vi "FOCUS_V42.vi"(9 "X-pixels":sgl=256.0, 11 "Run":bool) -> (0 "Retrace pixels":sgl, 10 "Pixel Clock (Hz)":sgl)   [LabVIEW 2010] (continued)
                            n2197 = To Unsigned Byte Integer(number=w3928) -> (unsigned 8bit integer=w3920:u8[])
                            n2198 = Add(x=w3895, y=w3899) -> (x+y=w3904:sgl[])
                            n2199 = To Unsigned Byte Integer(number=w3904) -> (unsigned 8bit integer=w3892:u8[])
                          }
                        }
                      }
                    }
                    n2200 = case shown="True" "Overlay Images" {
                      tunnel: w3665 -> [w4139 w4158]
                      tunnel: [w4139 w4141] -> w3812
                      tunnel: w3664 -> [w4138 w4160]
                      tunnel: [w4138 _] -> w3813
                      frame False {
                      }
                      frame True {
                        n2201 = To Word Integer(number=w4158) -> (16bit integer=w4159:i16[])
                        n2202 = Subtract(x=w4159, y=w4160) -> (x-y=w4140:i16[])
                        n2203 = Add(x=w4159, y=w4160) -> (x+y=w4154:i16[])
                        n2204 = Increment(x=w4154) -> (x+1=w4164:i16[])
                        n2205 = Divide(x=w4140, y=w4164) -> (x/y=w4163:dbl[])
                        n2206 = Absolute Value(x=w4140) -> (abs(x)=w4156:i16[])
                        n2207 = Multiply(x=w4163, y=u8 2) -> (x*y=w4161:dbl[])
                        n2208 = Round To Nearest(number=w4161) -> (nearest integer value=w4147:dbl[])
                        n2209 = Divide(x=w4156, y=2.0) -> (x/y=w4153:dbl[])
                        n2210 = Divide(x=w4154, y=2.0) -> (x/y=w4152:dbl[])
                        n2211 = Add(x=w4153, y=w4152) -> (x+y=w4150:dbl[])
                        n2212 = Divide(x=w4150, y=5.0) -> (x/y=w4149:dbl[])
                        n2213 = Round To Nearest(number=w4149) -> (nearest integer value=w4148:dbl[])
                        n2214 = Multiply(x=5.0 ("y"), y=w4148) -> (x*y=w4146:dbl[])
                        n2215 = Add(x=w4147, y=w4146) -> (x+y=w4145:dbl[])
                        n2216 = Subtract(x=w4145, y=2.0) -> (x-y=w4142:dbl[])
                        n2217 = To Unsigned Byte Integer(number=w4142) -> (unsigned 8bit integer=w4141:u8[])
                      }
                    }
                    n2218 = Greater Or Equal?(x=w3723, y=w3722) -> (x >= y?=w3657:bool)
                    n2219 = Sign(1:w3761) -> (0:w3760:i32)
                    n2220 = local write "Scan Backlock"(w3711) -> ()
                    n2221 = case shown="-1" w3760 {
                      tunnel: "Zoom" -> [_ w3965 w3970]
                      frame 0, Default {
                      }
                      frame 1 {
                        n2222 = Multiply(x=w3965, y=sgl 1.25) -> (x*y=w3963:sgl)
                        n2223 = local write "Zoom"(w3963) -> ()
                      }
                      frame -1 {
                        n2224 = Multiply(x=w3970, y=sgl 0.8) -> (x*y=w3966:sgl)
                        n2225 = Greater Or Equal?(x=w3966, y=sgl 0.28) -> (x >= y?=w3968:bool)
                        n2226 = case shown="True" w3968 {
                          tunnel: w3966 -> [_ w3971]
                          frame False {
                          }
                          frame True {
                            n2227 = local write "Zoom"(w3971) -> ()
                          }
                        }
                      }
                    }
                    n2228 = Not(x=w3680) -> (.not. x?=→"On?":bool)
                    n2229 = case shown="True" w3657 {
                      tunnel: w3769 -> [w3975 w4004]
                      tunnel: [w3975 w4003] -> w3768
                      tunnel: w3767 -> [w3976 w3982]
                      tunnel: [w3976 w3990] -> w3766
                      tunnel: w3718 -> [w3973 w3987]
                      tunnel: w3719 -> [w3974 w3984]
                      tunnel: [w3974 w3985] -> w3721
                      tunnel: [w3973 w3988] -> w3720
                      tunnel: [w3972 w3981] -> w3717
                      tunnel: w3716 -> [w3972 w3980]
                      tunnel: "scattering length [µm]" -> [_ w3977]
                      frame False {
                      }
                      frame True {
                        n2230 = local read "Sutter scale z"() -> (w3978:sgl)
                        n2231 = call "VISA MP-285 Get Z Position.vi"("Input: Duty Cluster"=w4004) -> ("Output: Z axis (microns)"=w4002:sgl, "Output: Duty Cluster"=w4003:T18, "error?"=w3981:bool)
                        n2232 = Multiply(x=w3978, y=w4002) -> (x*y=w3990:sgl)
                        n2233 = Equal?(x=TRUE, y="GetFirst") -> (x = y?=w3994:bool)
                        n2234 = Not Equal?(x="GetFirst", y=w3984) -> (x != y?=w3993:bool)
                        n2235 = Equal?(x=TRUE, y="GetLast") -> (x = y?=w3996:bool)
                        n2236 = Not Equal?(x="GetLast", y=w3987) -> (x != y?=w3998:bool)
                        n2237 = Subtract(x=w3990, y=w3982) -> (x-y=w3999:sgl)
                        n2238 = And(x=w3981, y=w3980) -> (x .and. y?=w3979:bool)
                        n2239 = Not Equal To 0?(x=w3999) -> (x != 0?=w4001:bool)
                        n2240 = Compound Arithmetic op=AND(w3994, w3993, w3979) -> (w3992:bool)
                        n2241 = Compound Arithmetic op=AND(w3979, w3996, w3998) -> (w3991:bool)
                        n2242 = Compound Arithmetic op=AND("IntensityAutomatic", w4001, w3979) -> (w3983:bool)
                        n2243 = case shown="True" w3992 {
                          tunnel: w3990 -> [_ w4007]
                          tunnel: "GetFirst" -> [_ w4006]
                          tunnel: [w4005 w4006] -> w3985
                          tunnel: w3984 -> [w4005 _]
                          frame False {
                          }
                          frame True {
                            "FirstPosition" <- w4007
                          }
                        }
                        n2244 = case shown="True" w3991 {
                          tunnel: w3990 -> [_ w4010]
                          tunnel: "GetLast" -> [_ w4009]
                          tunnel: [w4008 w4009] -> w3988
                          tunnel: w3987 -> [w4008 _]
                          frame False {
                          }
                          frame True {
                            "LastPosition" <- w4010
                          }
                        }
                        n2245 = case shown="True" w3983 {
                          tunnel: w3999 -> [_ w4014]
                          tunnel: w3990 -> [_ w4013]
                          tunnel: [w4011 w4013] -> _
                          tunnel: w3982 -> [w4011 _]
                          tunnel: w3977 -> [_ w4012]
                          frame False {
                          }
                          frame True {
                            n2246 = Divide(x=w4014, y=w4012) -> (x/y=w4021:sgl)
                            n2247 = local read "Intensity"() -> (w4019:sgl)
                            n2248 = Exponential(1:w4021) -> (0:w4020:sgl)
                            n2249 = local read "IntensityScaleMax"() -> (w4015:sgl)
                            n2250 = Multiply(x=w4019, y=w4020) -> (x*y=w4017:sgl)
                            n2251 = In Range and Coerce(upper limit=sgl 0.0, x=w4017, lower limit=w4015) -> (coerced(x)=w4016:sgl)  [unwired: 1 out]
                            n2252 = local write "Intensity"(w4016) -> ()
                          }
                        }
                      }
                    }
                    n2253 = Greater Or Equal?(x=w3811, y="Image Update [ms]") -> (x >= y?=w3809:bool)
                    n2254 = Greater Or Equal?(x=w3725, y=w3722) -> (x >= y?=w3653:bool)
                    n2255 = Replace Array Subset(array=w3770, new element=w3812, index (col)=w3725) -> (w3807:u8[][])  [unwired: 1 in]
                    n2256 = Replace Array Subset(array=w3777, new element=w3813, index (col)=w3725) -> (w3806:u8[][])  [unwired: 1 in]
                    n2257 = case shown="True" w3809 {
                      tunnel: [w4134 w4137] -> w3808
                      tunnel: w3794 -> [w4134 _]
                      tunnel: w3807 -> [_ w4136]
                      tunnel: w3806 -> [_ w4135]
                      frame False {
                      }
                      frame True {
                        n2258 = local write "Image 1"(w4136) -> ()
                        n2259 = local write "Image 2"(w4135) -> ()
                        n2260 = Tick Count (ms)() -> (millisecond timer value=w4137:u32)
                      }
                    }
                    n2261 = Unbundle By Name(w3742) -> ("status"=w3737:bool)
                    n2262 = case shown="False" w3653 {
                      tunnel: [w4037 i16 0] -> w3799
                      tunnel: w3725 -> [w4038 _]
                      frame False {
                        n2263 = Increment(x=w4038) -> (x+1=w4037:i16)
                      }
                      frame True {
                      }
                    }
                    n2264 = Unbundle By Name(w3741) -> ("status"=w3672:bool)
                    n2265 = case shown="False" w3657 {
                      tunnel: [w3956 i16 0] -> w3724
                      tunnel: w3723 -> [w3957 _]
                      frame False {
                        n2266 = Increment(x=w3957) -> (x+1=w3956:i16)
                      }
                      frame True {
                      }
                    }
                    n2267 = case shown="True" w3654 {
                      tunnel: w3665 -> [w3819 w3822]
                      tunnel: w3664 -> [w3816 w3821]
                      tunnel: w3663 -> [w3818 _]
                      tunnel: [w3817 w3820] -> w3660
                      frame True {
                        n2268 = Interleave 1D Arrays(w3816, w3819, w3818) -> (w3817:u8[])
                      }
                      frame False {
                        n2269 = Interleave 1D Arrays(w3822, w3821) -> (w3820:u8[])
                      }
                    }
                    n2270 = case shown="True" w3653 {
                      tunnel: w3662 -> [w3832 w3840]
                      tunnel: w3661 -> [w3831 w3839]
                      tunnel: w3660 -> [w3830 w3838]
                      tunnel: [w3829 w3837] -> w3659
                      tunnel: [w3828 w3836] -> w3658
                      frame True {
                        n2271 = Set File Position(offset (in bytes) (0)=768 ("pos offset (0)"), refnum=w3832, from (0:start)=enum16{"start", "end", "current"}."start" ("pos mode (0:2)"), error in=w3831) -> (refnum out=w3825:refnum<file>, error out=w3824:errorcluster)
                        n2272 = Write to Binary File(file (use dialog)=w3825, data=w3830, error in=w3824, 5:FALSE ("prepend array or string size? (T)")) -> (refnum out=w3829:refnum<file>, error out=w3828:errorcluster)  [unwired: 2 in, 1 out]
                      }
                      frame False {
                        n2273 = Set File Position(refnum=w3840, from (0:start)=enum16{"start", "end", "current"}."current" ("pos mode (0:2)"), error in=w3839) -> (refnum out=w3835:refnum<file>, error out=w3834:errorcluster)  [unwired: 1 in]
                        n2274 = Write to Binary File(file (use dialog)=w3835, data=w3838, error in=w3834, 5:FALSE ("prepend array or string size? (T)")) -> (refnum out=w3837:refnum<file>, error out=w3836:errorcluster)  [unwired: 2 in, 1 out]
                      }
                    }
                    n2275 = Unbundle By Name(w3712) -> ("status"=w3736:bool)
                    n2276 = local read "End experiment"() -> (w3732:bool)
                    n2277 = Unbundle By Name(w3738) -> ("status"=w3733:bool)
                    n2278 = Unbundle By Name(w3739) -> ("status"=w3734:bool)
                    n2279 = Unbundle By Name(w3740) -> ("status"=w3735:bool)
                    n2280 = Compound Arithmetic op=OR("stop 2", w3732, w3733, w3734, w3735, w3736, w3737, w3672) -> (w3730:bool)
                  }
                  n2281 = Not Equal?(x=w3574, y=w3573) -> (x != y?=→"IntDevUsed":bool)
                  n2282 = Close File(refnum=w3524, error in=w3523) -> ()  [unwired: 2 out]
                  n2283 = Unbundle(w3621) -> (w3599:sgl, w3598:sgl, w3597:sgl, "Zoom"=w3596:sgl, "x jog"=w3595:sgl, "y jog"=w3594:sgl, w3604:sgl, w3592:sgl)  [unwired: 5 out]
                  n2284 = call-poly <vilib>:"closeMouse.vi"("error in (no error)"=w3585, "device ID"=w3584) -> ("error out"=w3583:errorcluster)  [unwired: 8 in]
                  n2285 = call-poly <vilib>:"closeKeyboard.vi"("error in (no error)"=w3553, "device ID"=w3554) -> ("error out"=w3555:errorcluster)  [unwired: 8 in]
                  n2286 = call <vilib>:"Simple Error Handler.vi"("error in (no error)"=w3583) -> ()  [unwired: 4 in, 5 out]
                  n2287 = call <vilib>:"Simple Error Handler.vi"("error in (no error)"=w3555) -> ()  [unwired: 4 in, 5 out]
                  n2288 = local write "Zoom"(w3596) -> ()
                  n2289 = local write "x jog"(w3595) -> ()
                  n2290 = local write "y jog"(w3594) -> ()
                  n2291 = Multiply(x=w3604, y=sgl -1.0) -> (x*y=w3606:sgl)
                  n2292 = Subtract(x=w3606, y=sgl 360.0) -> (x-y=w3593:sgl)
                  n2293 = local write "Rotation"(w3593) -> ()
                  n2294 = flat-sequence {
                    tunnel: w3613 -> [w3651]
                    tunnel: [w3651] -> w3612
                    tunnel: w3578 -> [w3650]
                    frame #0 {
                      n2295 = Tick Count (ms)() -> (millisecond timer value=w3652:u32)
                      n2296 = local write "Parameters"(w3650) -> ()
                      n2297 = local write "stop"(w3652) -> ()
                    }
                  }
                  n2298 = Bundle(w3599, w3598, w3597, "Zoom"=w3596, "x jog"=w3595, "y jog"=w3594, w3593, w3592) -> (→"Scan Parameters":T32)  [unwired: 1 in]
                }
                frame 1 {
                  # "Iinner while loop runs for n loops, where n = number of averages.\nAll data acquired in this loop enters the average.\nThe z-step is activated each time this loop completes..\nThe outer while loop iterates m times, where m is total number of frames.\nControls are reset after the outer while loop completes.\nThe shutter is closed before and opened after each z-step."
                  # "Frame scan"
                  n2299 = flat-sequence {
                    tunnel: w4240 -> [w4249]
                    tunnel: [w4249] -> w4239
                    frame #0 {
                      n2300 = Tick Count (ms)() -> (millisecond timer value=→"start":u32)
                    }
                  }
                  n2301 = property on="Property Node" class="VI"() -> ("VI Path"=w4200:path)  [unwired: 2 in, 2 out]
                  n2302 = local read "x-step (um)"() -> (w4174:sgl)
                  n2303 = local read "y-step (um)"() -> (w4173:sgl)
                  n2304 = local read "z-step (um)"() -> (w4207:sgl)
                  n2305 = local read "z-positionstart (um)"() -> (w4175:sgl)
                  n2306 = Strip Path(path=w4200) -> (stripped path=w4199:path)  [unwired: 1 out]
                  n2307 = Equal To 0?(x=w4207) -> (x = 0?=w4170:bool)
                  n2308 = Equal To 0?(x=w4174) -> (x = 0?=w4171:bool)
                  n2309 = Equal To 0?(x=w4173) -> (x = 0?=w4172:bool)
                  n2310 = Initialize Array(u8 0 ("element"), w4218, w4217) -> (w4235:u8[][])
                  n2311 = Compound Arithmetic op=AND(w4171, w4172, w4170) -> (w4169:bool)
                  n2312 = Build Path(base path=w4199, name or relative path="Stack.tmp") -> (appended path=w4198:path)
                  n2313 = local write "FirstPosition"(w4175) -> ()
                  n2314 = call <vilib>:"Open_Create_Replace File.vi"("advisory dialog? (display:T)"=FALSE, "function (open:0)"=T8."create or replace", "file path"=w4198) -> ("error out"=w4191:errorcluster, "refnum"=w4193:refnum<file>)  [unwired: 5 in, 2 out]
                  n2315 = Set File Position(refnum=w4193, from (0:start)=enum16{"start", "end", "current"}."start" ("pos mode (rel. to end:1)"), error in=w4191) -> (refnum out=w4167:refnum<file>, error out=w4166:errorcluster)  [unwired: 1 in]
                  n2316 = Write to Binary File(file (use dialog)=w4167, data=w4189, error in=w4166, 5:FALSE ("prepend array or string size? (T)")) -> (refnum out=w4192:refnum<file>, error out=w4190:errorcluster)  [unwired: 2 in, 1 out]
                  n2317 = property on="Property Node" class="VI"() -> ("VI Path"=w4185:path)  [unwired: 2 in, 2 out]
                  n2318 = Strip Path(path=w4185) -> (stripped path=w4184:path)  [unwired: 1 out]
                  n2319 = Build Path(base path=w4184, name or relative path="EEG.tmp") -> (appended path=w4183:path)
                  n2320 = call <vilib>:"Open_Create_Replace File.vi"("advisory dialog? (display:T)"=FALSE, "function (open:0)"=T8."create or replace", "file path"=w4183) -> ("error out"=w4180:errorcluster, "refnum"=w4181:refnum<file>)  [unwired: 5 in, 2 out]
                  n2321 = while {
                    tunnel: [w4336] -> w4246
                    tunnel: [w4335] -> w4238
                    tunnel: w4245 -> [w4334]
                    tunnel: w4239 -> [w4333]
                    tunnel: w4244 -> [w4332]
                    tunnel: w4219 -> [w4258]
                    shift-right: [w4327] -> w4206
                    shift-left: w4235 -> [w4328]
                    shift-right: [w4325] -> w4205
                    shift-left: w4235 -> [w4326]
                    tunnel: [w4295] -> w4232
                    tunnel: w4234 -> [w4286]
                    tunnel: [w4293] -> w4231
                    tunnel: w4233 -> [w4287]
                    tunnel: w4176 -> [w4324]
                    tunnel: [w4323] -> w4220
                    tunnel: w4227 -> [w4322]
                    tunnel: w4225 -> [w4321]
                    tunnel: [w4320] -> w4226
                    tunnel: [w4319] -> w4224
                    tunnel: w4223 -> [w4292]
                    tunnel: w4222 -> [w4291]
                    tunnel: [w4317] -> w4212
                    tunnel: [w4316] -> w4221
                    tunnel: w4216 -> [w4310]
                    tunnel: w4215 -> [w4306]
                    tunnel: [w4309] -> w4214
                    tunnel: [w4308] -> w4213
                    tunnel: [w4284] -> w4211
                    tunnel: [w4298] -> w4209
                    tunnel: w4169 -> [w4271]
                    shift-right: [w4277] -> w4196
                    shift-left: w4192 -> [w4279]
                    shift-right: [w4276] -> w4195
                    shift-left: w4190 -> [w4278]
                    tunnel: w4188 -> [w4269]
                    shift-right: [w4266] -> w4179
                    shift-left: w4181 -> [w4268]
                    shift-right: [w4265] -> w4178
                    shift-left: w4180 -> [w4267]
                    tunnel: w4177 -> [w4264]
                    tunnel: w4168 -> [w4256]
                    i -> [w4284]
                    stop <- w4260 stop-if-true
                    w4272 = 0
                    n2322 = Equal To 0?(x=w4284) -> (x = 0?=w4311:bool)
                    n2323 = Greater Or Equal?(x=w4256, y=u16 3) -> (x >= y?=w4254:bool)
                    n2324 = Tick Count (ms)() -> (millisecond timer value=w4331:u32)
                    n2325 = Equal To 0?(x=w4284) -> (x = 0?=w4282:bool)
                    n2326 = Or(x=w4282, y=w4271) -> (x .or. y?=w4281:bool)
                    n2327 = case shown="False" w4281 {
                      tunnel: w4292 -> [w4347 w4356]
                      tunnel: [w4340 w4356] -> w4290
                      tunnel: w4291 -> [w4346 w4357]
                      tunnel: [w4339 w4357] -> w4289
                      tunnel: w4286 -> [w4344 w4354]
                      tunnel: w4287 -> [w4343 w4355]
                      tunnel: [w4338 w4355] -> w4288
                      tunnel: [w4337 w4354] -> w4285
                      frame False {
                        w4345 = TRUE ("data")
                        n2328 = local write "Shutter open"(w4345) -> ()
                        n2329 = call-poly <vilib>:"DAQmx Write (Digital Bool 1Line 1Point).vi"("task/channels in"=w4347, "data"=w4345, "error in"=w4346) -> ("task out"=w4342:refnum<k21>, "error out"=w4341:errorcluster)  [unwired: 10 in, 1 out]
                        n2330 = flat-sequence {
                          tunnel: w4344 -> [w4353]
                          tunnel: w4343 -> [w4352]
                          tunnel: w4342 -> [w4351]
                          tunnel: [w4351] -> w4340
                          tunnel: [w4350] -> w4339
                          tunnel: w4341 -> [w4350]
                          tunnel: [w4349] -> w4338
                          tunnel: [w4348] -> w4337
                          frame #0 {
                            n2331 = call <vilib>:"DAQmx Start Task.vi"("task/channels in"=w4353, "error in"=w4352) -> ("task out"=w4348:refnum<k21>, "error out"=w4349:errorcluster)  [unwired: 12 in]
                          }
                        }
                      }
                      frame True {
                      }
                    }
                    n2332 = Unbundle By Name(w4291) -> ("status"=w4305:bool)
                    n2333 = Unbundle By Name(w4306) -> ("status"=w4304:bool)
                    n2334 = Increment(x=w4284) -> (x+1=w4318:i32)
                    "#" <- w4318
                    n2335 = Compound Arithmetic op=OR(w4305, w4304) -> (w4303:bool)
                    n2336 = while {
                      tunnel: [w4486] -> w4336
                      tunnel: [w4488] -> w4335
                      tunnel: w4334 -> [w4510]
                      tunnel: w4333 -> [w4509]
                      shift-right: [w4516] -> w4275
                      shift-left: w4258 -> [w4515]
                      tunnel: w4332 -> [w4474]
                      shift-right: [w4517] -> w4274
                      shift-left: w4258 -> [w4518]
                      tunnel: [w4498] -> w4300
                      tunnel: [w4499] -> w4301
                      tunnel: ["z-step (um)"] -> w4283
                      tunnel: ["y-step (um)"] -> w4329
                      tunnel: ["x-step (um)"] -> w4330
                      shift-right: [w4531] -> _
                      shift-left: w4331 -> [w4532]
                      tunnel: w4311 -> [w4513]
                      tunnel: [w4457] -> w4296
                      tunnel: w4285 -> [w4457]
                      tunnel: [w4456] -> w4294
                      tunnel: w4288 -> [w4456]
                      tunnel: w4322 -> [w4512]
                      tunnel: w4321 -> [w4511]
                      tunnel: [w4505] -> w4320
                      tunnel: [w4476] -> w4319
                      tunnel: w4303 -> [w4497]
                      tunnel: [w4495] -> w4299
                      shift-right: [w4482] -> _
                      shift-left: w4272 -> [w4435]
                      shift-right: [w4481] -> _
                      shift-left: w4272 -> [w4434]
                      tunnel: w4269 -> [w4480]
                      shift-right: [w4467] -> w4266
                      shift-left: w4268 -> [w4470]
                      shift-right: [w4466] -> w4265
                      shift-left: w4267 -> [w4469]
                      tunnel: w4264 -> [w4451]
                      tunnel: w4256 -> [w4442]
                      shift-right: [w4433] -> w4257
                      shift-left: w4258 -> [w4436]
                      i -> [w4450]
                      stop <- w4496 stop-if-true
                      n2337 = local read "Scan Cut-Off (either end)"() -> (w4479:sgl)
                      n2338 = Equal To 0?(x="z-step (um)") -> (x = 0?=w4445:bool)
                      n2339 = Equal To 0?(x="y-step (um)") -> (x = 0?=w4446:bool)
                      n2340 = Equal To 0?(x="x-step (um)") -> (x = 0?=w4447:bool)
                      n2341 = Equal To 0?(x=w4450) -> (x = 0?=w4494:bool)
                      n2342 = call-poly <vilib>:"DAQmx Read (Analog 2D DBL NChan NSamp).vi"("task/channels in"=w4512, "number of samples per channel"=w4474, "error in"=w4511) -> ("task out"=w4505:refnum<k21>, "data"=w4475:dbl[][], "error out"=w4476:errorcluster)  [unwired: 10 in]
                      n2343 = Compound Arithmetic op=AND(w4445, w4446, w4447) -> (w4444:bool)
                      n2344 = local read "End experiment"() -> (w4499:bool)
                      n2345 = local read "Cusp Delay"() -> (w4477:sgl)
                      n2346 = case shown="True" w4444 {
                        tunnel: w4513 -> [_ w4640]
                        tunnel: w4494 -> [w4637 w4639]
                        tunnel: [w4637 w4638] -> w4493
                        frame False {
                        }
                        frame True {
                          n2347 = And(x=w4639, y=w4640) -> (x .and. y?=w4638:bool)
                        }
                      }
                      n2348 = case shown="False" w4493 {
                        tunnel: w4474 -> [w4641 w4647]
                        tunnel: [w4641 w4643] -> w4458
                        tunnel: w4479 -> [w4642 w4646]
                        tunnel: [w4642 w4645] -> w4503
                        tunnel: w4480 -> [_ w4644]
                        frame False {
                        }
                        frame True {
                          n2349 = Add(x=w4647, y=w4644) -> (x+y=w4643:sgl)
                          n2350 = Add(x=w4646, y=w4644) -> (x+y=w4645:sgl)
                        }
                      }
                      n2351 = call-poly <vilib>:"DAQmx Read (Digital 1D U32 1Chan NSamp).vi"("task/channels in"=w4510, "number of samples per channel"=w4458, "error in"=w4509) -> ("task out"=w4487:refnum<k21>, "data"=w4461:u32[], "error out"=w4489:errorcluster)  [unwired: 10 in]
                      n2352 = local read "X-pixels"() -> (w4508:sgl)
                      n2353 = local read "Overlay Images"() -> (w4514:bool)
                      n2354 = local read "stop 2"() -> (w4498:bool)
                      n2355 = Unbundle By Name(w4489) -> ("status"=w4501:bool)
                      n2356 = Unbundle By Name(w4456) -> ("status"=w4502:bool)
                      n2357 = Add(x=w4503, y=w4477) -> (x+y=w4478:sgl)
                      n2358 = local read "total y pixels"() -> (w4462:sgl)
                      n2359 = case shown="1" w4451 {
                        tunnel: w4450 -> [_ w4625]
                        tunnel: w4461 -> [w4620 w4623]
                        tunnel: [w4620 w4622] -> w4459
                        frame 0, Default {
                        }
                        frame 1 {
                          n2360 = local read "Shift"() -> (w4621:sgl)
                          n2361 = call "testoddevenFOCUS.vi"("Numeric"=w4625) -> ("Boolean"=w4624:bool)
                          n2362 = case shown="True" w4624 {
                            tunnel: w4623 -> [w4627 w4630]
                            tunnel: [w4626 w4628] -> w4622
                            tunnel: w4621 -> [_ w4629]
                            frame False {
                              n2363 = Reverse 1D Array(array=w4627) -> (reversed array=w4626:u32[])
                            }
                            frame True {
                              n2364 = Rotate 1D Array(1:w4630, 2:w4629) -> (0:w4628:u32[])
                            }
                          }
                        }
                      }
                      n2365 = Array Subset "Extract DI0"(array=w4459, index=w4478, length=w4508) -> (w4460:u32[])
                      n2366 = Split Number(x=w4460) -> (hi(x)=w4506:u16[], lo(x)=w4443:u16[])
                      n2367 = property class="DAQmx Read"(reference=w4487, error in=w4489) -> (reference out=w4486:refnum<k21>, error out=w4488:errorcluster, "Status:Available Samples Per Channel"=w4485:u32)
                      n2368 = case shown="0, Default" w4442 {
                        tunnel: w4506 -> [w4542 w4547 w4552 w4557 w4562 w4567]
                        tunnel: [w4541 w4546 w4549 w4556 w4561 w4564] -> w4455
                        tunnel: [w4539 w4544 w4551 w4554 w4559 w4566] -> w4453
                        tunnel: w4443 -> [w4540 w4545 w4550 w4555 w4560 w4565]
                        tunnel: [w4538 w4543 w4548 w4553 w4558 w4563] -> w4432
                        frame 0, Default {
                          n2369 = Split Number(x=w4542) -> (hi(x)=w4541:u8[], lo(x)=w4539:u8[])
                          n2370 = Split Number(x=w4540) -> (lo(x)=w4538:u8[])  [unwired: 1 out]
                        }
                        frame 1 {
                          n2371 = Split Number(x=w4547) -> (hi(x)=w4546:u8[], lo(x)=w4543:u8[])
                          n2372 = Split Number(x=w4545) -> (lo(x)=w4544:u8[])  [unwired: 1 out]
                        }
                        frame 2 {
                          n2373 = Split Number(x=w4552) -> (hi(x)=w4548:u8[], lo(x)=w4551:u8[])
                          n2374 = Split Number(x=w4550) -> (lo(x)=w4549:u8[])  [unwired: 1 out]
                        }
                        frame 3 {
                          n2375 = Split Number(x=w4557) -> (hi(x)=w4556:u8[], lo(x)=w4554:u8[])
                          n2376 = Split Number(x=w4555) -> (lo(x)=w4553:u8[])  [unwired: 1 out]
                        }
                        frame 4 {
                          n2377 = Split Number(x=w4562) -> (hi(x)=w4561:u8[], lo(x)=w4558:u8[])
                          n2378 = Split Number(x=w4560) -> (lo(x)=w4559:u8[])  [unwired: 1 out]
                        }
                        frame 5 {
                          n2379 = Split Number(x=w4567) -> (hi(x)=w4563:u8[], lo(x)=w4566:u8[])
                          n2380 = Split Number(x=w4565) -> (lo(x)=w4564:u8[])  [unwired: 1 out]
                        }
                      }
                      n2381 = Multiply(x="Averaging", y=w4462) -> (x*y=w4535:sgl)
                      n2382 = Increment(x=w4450) -> (x+1=w4507:i32)
                      n2383 = Equal?(x=w4507, y=w4535) -> (x = y?=w4500:bool)
                      n2384 = Compound Arithmetic op=OR(w4502, w4501) -> (w4495:bool)
                      n2385 = Transpose 2D Array(2D array=w4475) -> (transposed array=w4468:dbl[][])
                      n2386 = Divide(x=w4507, y=w4462) -> (x/y=w4464:sgl)
                      n2387 = local write "Scan Backlock"(w4485) -> ()
                      n2388 = Round Toward +Infinity(x=w4464) -> (ceil(x): smallest int >= x=w4463:sgl)
                      "#" <- w4463
                      n2389 = case shown="1" w4451 {
                        tunnel: w4455 -> [w4570 w4577]
                        tunnel: [w4570 w4576] -> w4454
                        tunnel: w4450 -> [_ w4579]
                        tunnel: w4453 -> [w4569 w4574]
                        tunnel: [w4569 w4573] -> w4452
                        tunnel: w4432 -> [w4568 w4572]
                        tunnel: [w4568 w4571] -> w4431
                        frame 0, Default {
                        }
                        frame 1 {
                          n2390 = local read "Shift"() -> (w4575:sgl)
                          n2391 = call "testoddevenFOCUS.vi"("Numeric"=w4579) -> ("Boolean"=w4578:bool)
                          n2392 = case shown="True" w4578 {
                            tunnel: w4577 -> [w4582 w4609]
                            tunnel: [w4582 w4611] -> w4576
                            tunnel: w4575 -> [_ w4585]
                            tunnel: w4574 -> [w4581 w4597]
                            tunnel: [w4581 w4596] -> w4573
                            tunnel: w4572 -> [w4580 w4584]
                            tunnel: [w4580 w4583] -> w4571
                            frame False {
                            }
                            frame True {
                              n2393 = Round Toward -Infinity(1:w4585) -> (0:w4601:sgl)
                              n2394 = Round Toward -Infinity(1:w4585) -> (0:w4616:sgl)
                              n2395 = Round Toward -Infinity(1:w4585) -> (0:w4592:sgl)
                              n2396 = To Word Integer(number=w4597) -> (16bit integer=w4607:i16[])
                              n2397 = To Word Integer(number=w4609) -> (16bit integer=w4608:i16[])
                              n2398 = To Word Integer(number=w4584) -> (16bit integer=w4586:i16[])
                              n2399 = Array Subset(array=w4607, index=1) -> (w4600:i16[])  [unwired: 1 in]
                              n2400 = Array Subset(array=w4608, index=1) -> (w4617:i16[])  [unwired: 1 in]
                              n2401 = Array Subset(array=w4586, index=1) -> (w4593:i16[])  [unwired: 1 in]
                              n2402 = Subtract(x=w4585, y=w4601) -> (x-y=w4602:sgl)
                              n2403 = Subtract(x=w4585, y=w4616) -> (x-y=w4615:sgl)
                              n2404 = Subtract(x=w4585, y=w4592) -> (x-y=w4591:sgl)
                              n2405 = Subtract(x=w4607, y=w4600) -> (x-y=w4604:i16[])
                              n2406 = Subtract(x=w4608, y=w4617) -> (x-y=w4613:i16[])
                              n2407 = Subtract(x=w4586, y=w4593) -> (x-y=w4589:i16[])
                              n2408 = Build Array (concatenate)(0 ("index"), w4604) -> (w4605:i32[])
                              n2409 = Build Array (concatenate)(0 ("index"), w4613) -> (w4612:i32[])
                              n2410 = Build Array (concatenate)(0 ("index"), w4589) -> (w4588:i32[])
                              n2411 = Multiply(x=w4602, y=w4605) -> (x*y=w4603:sgl[])
                              n2412 = Multiply(x=w4615, y=w4612) -> (x*y=w4614:sgl[])
                              n2413 = Multiply(x=w4591, y=w4588) -> (x*y=w4590:sgl[])
                              n2414 = Add(x=w4607, y=w4603) -> (x+y=w4598:sgl[])
                              n2415 = To Unsigned Byte Integer(number=w4598) -> (unsigned 8bit integer=w4596:u8[])
                              n2416 = Add(x=w4608, y=w4614) -> (x+y=w4619:sgl[])
                              n2417 = To Unsigned Byte Integer(number=w4619) -> (unsigned 8bit integer=w4611:u8[])
                              n2418 = Add(x=w4586, y=w4590) -> (x+y=w4595:sgl[])
                              n2419 = To Unsigned Byte Integer(number=w4595) -> (unsigned 8bit integer=w4583:u8[])
                            }
                          }
                        }
                      }
                      n2420 = case shown="True" w4514 {
                        tunnel: w4454 -> [w4653 w4656]
                        tunnel: [w4653 w4654] -> w4520
                        tunnel: w4452 -> [w4652 w4655]
                        tunnel: [w4652 _] -> w4519
                        frame False {
                        }
                        frame True {
                          n2421 = To Word Integer(number=w4656) -> (16bit integer=w4661:i16[])
                          n2422 = Subtract(x=w4661, y=w4655) -> (x-y=w4662:i16[])
                          n2423 = Add(x=w4661, y=w4655) -> (x+y=w4666:i16[])
                          n2424 = Increment(x=w4666) -> (x+1=w4657:i16[])
                          n2425 = Divide(x=w4662, y=w4657) -> (x/y=w4658:dbl[])
                          n2426 = Absolute Value(x=w4662) -> (abs(x)=w4664:i16[])
                          n2427 = Multiply(x=w4658, y=u8 2) -> (x*y=w4660:dbl[])
                          n2428 = Round To Nearest(number=w4660) -> (nearest integer value=w4673:dbl[])
                          n2429 = Divide(x=w4664, y=2.0) -> (x/y=w4667:dbl[])
                          n2430 = Divide(x=w4666, y=2.0) -> (x/y=w4668:dbl[])
                          n2431 = Add(x=w4667, y=w4668) -> (x+y=w4670:dbl[])
                          n2432 = Divide(x=w4670, y=5.0) -> (x/y=w4671:dbl[])
                          n2433 = Round To Nearest(number=w4671) -> (nearest integer value=w4672:dbl[])
                          n2434 = Multiply(x=5.0 ("y"), y=w4672) -> (x*y=w4674:dbl[])
                          n2435 = Add(x=w4673, y=w4674) -> (x+y=w4675:dbl[])
                          n2436 = Subtract(x=w4675, y=2.0) -> (x-y=w4678:dbl[])
                          n2437 = To Unsigned Byte Integer(number=w4678) -> (unsigned 8bit integer=w4654:u8[])
                        }
                      }
                      n2438 = Compound Arithmetic op=OR(w4495, w4500, w4499, w4498, w4497) -> (w4496:bool)
                      n2439 = Subtract(x=w4464, y=w4463) -> (x-y=w4491:sgl)
                      n2440 = Equal To 0?(x=w4491) -> (x = 0?=w4465:bool)
                      n2441 = Tick Count (ms)() -> (millisecond timer value=w4534:u32)
                      n2442 = local read "total y pixels"() -> (w4537:sgl)
                      n2443 = while {
                        tunnel: w4537 -> [w4681]
                        shift-right: [w4682] -> _
                        shift-left: w4450 -> [w4680]
                        tunnel: [w4680] -> _
                        tunnel: [w4679] -> _
                        i -> [w4679]
                        stop <- w4683 stop-if-true
                        n2444 = Subtract(x=w4680, y=w4681) -> (x-y=w4682:sgl)
                        n2445 = Less?(x=w4680, y=w4681) -> (x < y?=w4683:bool)
                      }
                      n2446 = Decrement(x=w4462) -> (x-1=w4484:sgl)
                      n2447 = Index Array(array=w4468, index (col)=3 ("disabled index (col)")) -> (element=w4473:dbl[])  [unwired: 1 in]
                      n2448 = Subtract(x=w4534, y=w4532) -> (x-y=w4533:u32)
                      n2449 = Set File Position(refnum=w4470, from (0:start)=enum16{"start", "end", "current"}."current" ("pos mode (0:2)"), error in=w4469) -> (refnum out=w4430:refnum<file>, error out=w4429:errorcluster)  [unwired: 1 in]
                      n2450 = Greater Or Equal?(x=w4435, y=w4484) -> (x >= y?=w4483:bool)
                      n2451 = Write to Binary File(file (use dialog)=w4430, data=w4473, error in=w4429, 5:FALSE ("prepend array or string size? (T)")) -> (refnum out=w4467:refnum<file>, error out=w4466:errorcluster)  [unwired: 2 in, 1 out]
                      n2452 = local read "Image Update [ms]"() -> (w4504:u32)
                      n2453 = Index Array(array=w4515, index (col)=w4435) -> (element=w4521:u8[])  [unwired: 1 in]
                      n2454 = case shown="True" w4483 {
                        tunnel: [w4632 i16 0] -> w4482
                        tunnel: w4435 -> [w4633 _]
                        tunnel: w4434 -> [w4631 w4635]
                        tunnel: [w4631 w4634] -> w4481
                        frame False {
                          n2455 = Increment(x=w4633) -> (x+1=w4632:i32)
                        }
                        frame True {
                          n2456 = Increment(x=w4635) -> (x+1=w4634:i32)
                        }
                      }
                      n2457 = Multiply(x=w4521, y=w4434) -> (x*y=w4522:i32[])
                      n2458 = Add(x=w4522, y=w4520) -> (x+y=w4524:i32[])
                      n2459 = Index Array(array=w4518, index (col)=w4435) -> (element=w4530:u8[])  [unwired: 1 in]
                      n2460 = Greater Or Equal?(x=w4533, y=w4504) -> (x >= y?=w4490:bool)
                      n2461 = Increment(x=w4434) -> (x+1=w4523:i32)
                      n2462 = Multiply(x=w4530, y=w4434) -> (x*y=w4529:i32[])
                      n2463 = Divide(x=w4524, y=w4523) -> (x/y=w4525:dbl[])
                      n2464 = Add(x=w4529, y=w4519) -> (x+y=w4527:i32[])
                      n2465 = Increment(x=w4434) -> (x+1=w4528:i32)
                      n2466 = Index Array(array=w4436, index (col)=w4435) -> (element=w4437:u8[])  [unwired: 1 in]
                      n2467 = Replace Array Subset(array=w4515, new element=w4525, index (col)=w4435) -> (w4516:u8[][])  [unwired: 1 in]
                      n2468 = Or(x=w4465, y=w4490) -> ()  [unwired: 1 out]
                      n2469 = Divide(x=w4527, y=w4528) -> (x/y=w4526:dbl[])
                      n2470 = Multiply(x=w4437, y=w4434) -> (x*y=w4438:i32[])
                      n2471 = Add(x=w4438, y=w4431) -> (x+y=w4440:i32[])
                      n2472 = Increment(x=w4434) -> (x+1=w4439:i32)
                      n2473 = Replace Array Subset(array=w4518, new element=w4526, index (col)=w4435) -> (w4517:u8[][])  [unwired: 1 in]
                      n2474 = Divide(x=w4440, y=w4439) -> (x/y=w4441:dbl[])
                      n2475 = case shown="True" w4465 {
                        tunnel: [w4648 w4651] -> w4531
                        tunnel: w4532 -> [w4648 _]
                        tunnel: w4516 -> [_ w4650]
                        tunnel: w4517 -> [_ w4649]
                        frame False {
                        }
                        frame True {
                          n2476 = local write "Image 2"(w4649) -> ()
                          n2477 = local write "Image 1"(w4650) -> ()
                          n2478 = Tick Count (ms)() -> (millisecond timer value=w4651:u32)
                        }
                      }
                      n2479 = Replace Array Subset(array=w4436, new element=w4441, index (col)=w4435) -> (w4433:u8[][])  [unwired: 1 in]
                    }
                    n2480 = Not(x="Go further?") -> (.not. x?=w4263:bool)
                    n2481 = Equal?(x="Number of frames", y=w4318) -> (x = y?=w4302:bool)
                    n2482 = Compound Arithmetic op=OR(w4299, w4300, w4301, w4302, w4303) -> (w4270:bool)
                    n2483 = Or(x=w4270, y=w4271) -> (x .or. y?=w4261:bool)
                    n2484 = Select(t=w4263, s="Go further?", f=w4261) -> (s? t:f=w4259:bool)
                    n2485 = local read "IntensityAutomatic"() -> (w4297:bool)
                    n2486 = case shown="False" w4259 {
                      tunnel: [w4369 w4419] -> w4260
                      tunnel: w4330 -> [w4364 _]
                      tunnel: w4329 -> [w4363 _]
                      tunnel: w4283 -> [w4362 _]
                      tunnel: w4324 -> [w4388 w4427]
                      tunnel: [w4387 w4427] -> w4323
                      tunnel: w4290 -> [w4373 w4424]
                      tunnel: w4289 -> [w4372 w4423]
                      tunnel: [w4371 w4424] -> w4317
                      tunnel: [w4370 w4423] -> w4316
                      tunnel: w4310 -> [w4383 w4426]
                      tunnel: w4306 -> [w4382 w4425]
                      tunnel: [w4381 w4426] -> w4309
                      tunnel: [w4380 w4425] -> w4308
                      tunnel: [w4379 w4422] -> w4298
                      tunnel: w4297 -> [w4378 _]
                      tunnel: w4296 -> [w4376 w4421]
                      tunnel: w4294 -> [w4377 w4420]
                      tunnel: [w4375 w4421] -> w4295
                      tunnel: [w4374 w4420] -> w4293
                      tunnel: w4270 -> [w4369 w4419]
                      frame False {
                        n2487 = local read "Sutter scale x"() -> (w4365:sgl)
                        n2488 = local read "Sutter scale y"() -> (w4366:sgl)
                        n2489 = local read "Sutter scale z"() -> (w4367:sgl)
                        n2490 = case shown="True" w4378 {
                          tunnel: w4383 -> [w4404 w4413]
                          tunnel: w4382 -> [w4403 w4412]
                          tunnel: [w4404 w4411] -> w4381
                          tunnel: [w4403 w4410] -> w4380
                          tunnel: [w4402 w4405] -> w4379
                          tunnel: w4362 -> [_ w4406]
                          frame False {
                            n2491 = local read "Intensity"() -> (w4402:sgl)
                          }
                          frame True {
                            n2492 = local read "scattering length [µm]"() -> (w4416:sgl)
                            n2493 = Divide(x=w4406, y=w4416) -> (x/y=w4418:sgl)
                            n2494 = Exponential(1:w4418) -> (0:w4417:sgl)
                            n2495 = local read "Intensity"() -> (w4415:sgl)
                            n2496 = local read "IntensityScaleMax"() -> (w4407:sgl)
                            n2497 = Multiply(x=w4415, y=w4417) -> (x*y=w4408:sgl)
                            n2498 = In Range and Coerce(upper limit=sgl 0.0, x=w4408, lower limit=w4407) -> (coerced(x)=w4405:sgl)  [unwired: 1 out]
                            n2499 = local write "Intensity"(w4405) -> ()
                            n2500 = Build Array(sgl 0.0 ("element"), w4405) -> ()  [unwired: 1 out]
                            n2501 = call-poly <vilib>:"DAQmx Write (Analog DBL 1Chan 1Samp).vi"("task/channels in"=w4413, "data"=w4405, "error in"=w4412) -> ("task out"=w4411:refnum<k21>, "error out"=w4410:errorcluster)  [unwired: 10 in, 1 out]
                          }
                        }
                        n2502 = Divide(x=w4364, y=w4365) -> (x/y=w4384:sgl)
                        n2503 = Divide(x=w4363, y=w4366) -> (x/y=w4385:sgl)
                        n2504 = Divide(x=w4362, y=w4367) -> (x/y=w4386:sgl)
                        n2505 = Not Equal To 0?(x=w4362) -> (x != 0?=w4360:bool)
                        n2506 = Not Equal To 0?(x=w4363) -> (x != 0?=w4361:bool)
                        n2507 = Not Equal To 0?(x=w4364) -> (x != 0?=w4359:bool)
                        n2508 = call "VISA MP-285 Step.vi"("Input: Duty Cluster"=w4388, "Input: Delta Z axis (microns)"=w4386, "Input: Delta Y axis (microns)"=w4385, "Input: Delta X axis (microns)"=w4384) -> ("Output: Duty Cluster"=w4387:T18)  [unwired: 3 out]
                        n2509 = Wait (ms)(milliseconds to wait=u32 50) -> ()  [unwired: 1 out]
                        n2510 = Compound Arithmetic op=OR(w4360, w4361, w4359) -> (w4358:bool)
                        n2511 = case shown="True" w4358 {
                          tunnel: w4377 -> [w4391 w4401]
                          tunnel: w4376 -> [w4392 w4400]
                          tunnel: [w4392 w4399] -> w4375
                          tunnel: [w4391 w4398] -> w4374
                          tunnel: w4373 -> [w4390 w4397]
                          tunnel: w4372 -> [w4389 w4396]
                          tunnel: [w4390 w4395] -> w4371
                          tunnel: [w4389 w4394] -> w4370
                          frame False {
                          }
                          frame True {
                            w4393 = FALSE ("data")
                            n2512 = call <vilib>:"DAQmx Stop Task.vi"("task/channels in"=w4400, "error in"=w4401) -> ("task out"=w4399:refnum<k21>, "error out"=w4398:errorcluster)  [unwired: 12 in]
                            n2513 = local write "Shutter open"(w4393) -> ()
                            n2514 = call-poly <vilib>:"DAQmx Write (Digital Bool 1Line 1Point).vi"("task/channels in"=w4397, "data"=w4393, "error in"=w4396) -> ("task out"=w4395:refnum<k21>, "error out"=w4394:errorcluster)  [unwired: 10 in, 1 out]
                          }
                        }
                      }
                      frame True {
                        n2515 = local read "Intensity"() -> (w4422:sgl)
                      }
                    }
                    "frame scan finished?" <- w4260
                    n2516 = call "ConvertImagesDataFOCUS.vi"("Save mode"=w4254, "Image3"=w4257, "Image2"=w4274, "Image1"=w4275) -> ("Data"=w4273:u8[])
                    n2517 = Set File Position(refnum=w4279, from (0:start)=enum16{"start", "end", "current"}."current" ("pos mode (0:2)"), error in=w4278) -> (refnum out=w4253:refnum<file>, error out=w4252:errorcluster)  [unwired: 1 in]
                    n2518 = local read "Y-lines"() -> (w4313:sgl)
                    n2519 = Write to Binary File(file (use dialog)=w4253, data=w4273, error in=w4252, 5:FALSE ("prepend array or string size? (T)")) -> (refnum out=w4277:refnum<file>, error out=w4276:errorcluster)  [unwired: 2 in, 1 out]
                    n2520 = Multiply(x=w4313, y=w4284) -> (x*y=w4312:sgl)
                    n2521 = Replace Array Subset(array=w4326, new element=w4274, index (row)=0 ("disabled index (row)"), index (col)=w4312) -> (w4325:u8[][])
                    n2522 = Replace Array Subset(array=w4328, new element=w4275, index (row)=0 ("disabled index (row)"), index (col)=w4312) -> (w4327:u8[][])
                  }
                  n2523 = local read "Intensity"() -> (w4210:sgl)
                  n2524 = Not Equal?(x=w4209, y=w4210) -> (x != y?=w4208:bool)
                  n2525 = local write "IntDevUsed"(w4208) -> ()
                  n2526 = Close File(refnum=w4196, error in=w4195) -> ()  [unwired: 2 out]
                  n2527 = Close File(refnum=w4179, error in=w4178) -> ()  [unwired: 2 out]
                  n2528 = flat-sequence {
                    tunnel: w4238 -> [w4247]
                    tunnel: [w4247] -> w4237
                    frame #0 {
                      n2529 = Tick Count (ms)() -> (millisecond timer value=→"stop":u32)
                    }
                  }
                }
                frame 2 {
                  # "Straight line scan"
                  n2530 = flat-sequence {
                    tunnel: w4733 -> [w4743]
                    tunnel: [w4743] -> w4732
                    frame #0 {
                      n2531 = Tick Count (ms)() -> (millisecond timer value=w4744:u32)
                      n2532 = local write "start"(w4744) -> ()
                    }
                  }
                  n2533 = Decrement(x=w4712) -> (x-1=w4711:sgl)
                  n2534 = Unbundle By Name(w4718) -> ("status"=w4716:bool)
                  n2535 = property on="Image 1" class="IntGraph (strict)"("Y Scale.Range:Maximum"=w4711) -> ()  [unwired: 2 in, 2 out]
                  n2536 = Initialize Array(u8 0 ("element"), w4712, w4713) -> (w4714:u8[][])
                  n2537 = Greater Or Equal?(x=w4689, y=u16 3) -> (x >= y?=w4687:bool)
                  n2538 = property on="Property Node" class="VI"() -> ("VI Path"=w4703:path)  [unwired: 2 in, 2 out]
                  n2539 = Unbundle By Name(w4719) -> ("status"=w4717:bool)
                  n2540 = Tick Count (ms)() -> (millisecond timer value=w4734:u32)
                  n2541 = property on="Image 2" class="IntGraph (strict)"("Y Scale.Range:Maximum"=w4711) -> ()  [unwired: 2 in, 2 out]
                  n2542 = Strip Path(path=w4703) -> (stripped path=w4702:path)  [unwired: 1 out]
                  n2543 = Build Path(base path=w4702, name or relative path="Stack.tmp") -> (appended path=w4701:path)
                  n2544 = call <vilib>:"Open_Create_Replace File.vi"("advisory dialog? (display:T)"=FALSE, "function (open:0)"=T8."create or replace", "file path"=w4701) -> ("error out"=w4694:errorcluster, "refnum"=w4696:refnum<file>)  [unwired: 5 in, 2 out]
                  n2545 = Set File Position(refnum=w4696, from (0:start)=enum16{"start", "end", "current"}."start" ("pos mode (rel. to end:1)"), error in=w4694) -> (refnum out=w4686:refnum<file>, error out=w4685:errorcluster)  [unwired: 1 in]
                  n2546 = Write to Binary File(file (use dialog)=w4686, data=w4692, error in=w4685, 5:FALSE ("prepend array or string size? (T)")) -> (refnum out=w4695:refnum<file>, error out=w4693:errorcluster)  [unwired: 2 in, 1 out]
                  n2547 = while {
                    tunnel: [w4769] -> w4736
                    tunnel: [w4767] -> w4731
                    tunnel: w4737 -> [w4795]
                    tunnel: w4732 -> [w4785]
                    shift-right: [w4814] -> w4710
                    shift-left: w4714 -> [w4816]
                    tunnel: w4738 -> [w4800]
                    shift-right: [w4813] -> w4709
                    shift-left: w4714 -> [w4815]
                    shift-right: [w4807] -> _
                    shift-left: w4734 -> [w4808]
                    tunnel: w4726 -> [w4796]
                    tunnel: w4725 -> [w4786]
                    tunnel: [w4796] -> w4724
                    tunnel: [w4786] -> w4723
                    tunnel: [w4791] -> w4720
                    tunnel: w4717 -> [w4784]
                    tunnel: w4716 -> [w4781]
                    tunnel: w4713 -> [w4776]
                    shift-right: [w4772] -> w4698
                    shift-left: w4695 -> [w4774]
                    shift-right: [w4771] -> w4699
                    shift-left: w4693 -> [w4773]
                    tunnel: w4691 -> [w4765]
                    tunnel: w4690 -> [w4761]
                    tunnel: w4689 -> [w4759]
                    tunnel: w4687 -> [w4750]
                    i -> [w4762]
                    stop <- w4777 stop-if-true
                    n2548 = local read "Scan Cut-Off (either end)"() -> (w4798:sgl)
                    n2549 = Equal To 0?(x=w4762) -> (x = 0?=w4799:bool)
                    n2550 = Unbundle By Name(w4785) -> ("status"=w4782:bool)
                    n2551 = case shown="False" w4799 {
                      tunnel: w4800 -> [w4918 w4923]
                      tunnel: [w4918 w4922] -> w4794
                      tunnel: w4798 -> [w4917 w4921]
                      tunnel: [w4917 w4920] -> w4787
                      tunnel: w4765 -> [_ w4919]
                      frame False {
                      }
                      frame True {
                        n2552 = Add(x=w4923, y=w4919) -> (x+y=w4922:sgl)
                        n2553 = Add(x=w4921, y=w4919) -> (x+y=w4920:sgl)
                      }
                    }
                    n2554 = call-poly <vilib>:"DAQmx Read (Digital 1D U32 1Chan NSamp).vi"("task/channels in"=w4795, "number of samples per channel"=w4794, "error in"=w4785) -> ("task out"=w4770:refnum<k21>, "data"=w4764:u32[], "error out"=w4768:errorcluster)  [unwired: 10 in]
                    n2555 = case shown="1" w4761 {
                      tunnel: w4762 -> [_ w4911]
                      tunnel: w4764 -> [w4906 w4909]
                      tunnel: [w4906 w4908] -> w4763
                      frame 0, Default {
                      }
                      frame 1 {
                        n2556 = local read "Shift"() -> (w4907:sgl)
                        n2557 = call "testoddevenFOCUS.vi"("Numeric"=w4911) -> ("Boolean"=w4910:bool)
                        n2558 = case shown="False" w4910 {
                          tunnel: w4909 -> [w4913 w4916]
                          tunnel: [w4912 w4914] -> w4908
                          tunnel: w4907 -> [_ w4915]
                          frame False {
                            n2559 = Reverse 1D Array(array=w4913) -> (reversed array=w4912:u32[])
                          }
                          frame True {
                            n2560 = Rotate 1D Array(1:w4916, 2:w4915) -> (0:w4914:u32[])
                          }
                        }
                      }
                    }
                    n2561 = local read "Cusp Delay"() -> (w4789:sgl)
                    n2562 = local read "X-pixels"() -> (w4790:sgl)
                    n2563 = Add(x=w4787, y=w4789) -> (x+y=w4788:sgl)
                    n2564 = local read "End experiment"() -> (w4779:bool)
                    n2565 = Unbundle By Name(w4786) -> ("status"=w4783:bool)
